vi "RemoveEchoSerial.vi"(9 "message":string, 11 "String in":string) -> (3 "String out":string)   [LabVIEW 2018]
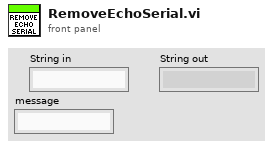
[diagram p1: front panel]
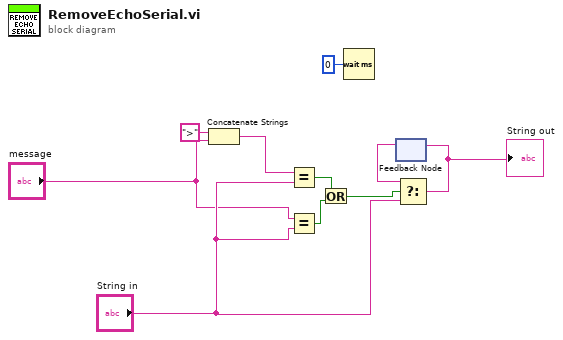
[diagram p0: block diagram]
diagram:
  n1 = Concatenate Strings(">" ("string"), "message") -> (w8:string)
  n2 = Equal?(x=w8, y="String in") -> (x = y?=w6:bool)
  n3 = Equal?(x="message", y="String in") -> (x = y?=w4:bool)
  n4 = Or(x=w6, y=w4) -> (x .or. y?=w5:bool)
  n5 = Wait (ms)(milliseconds to wait=u32 0) -> ()  [unwired: 1 out]
  n6 = feedback #1() -> (w9:string)  [unwired: 1 in]
  n7 = Select(t=w9, s=w5, f="String in") -> (s? t:f=w10:string)
  "String out" <- w10
  n8 = feedback-in #1(w10) -> ()
